vi "Log to File.vi"(8 "error in":errorcluster, 10 "Waveform Graph":dbl[](graph), 11 "Log File Path":path) -> (0 "error out":errorcluster)   [LabVIEW 2015]
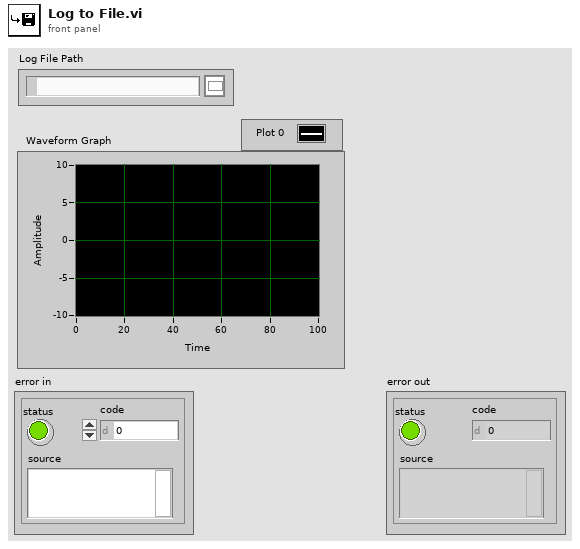
[diagram p1: front panel]
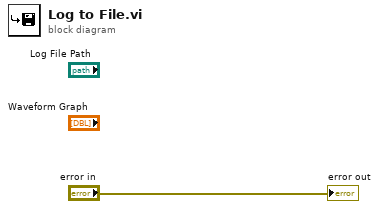
[diagram p0: block diagram]
diagram:
  "error out" <- "error in"
